vi "Target Detection.vi"(0 "Camera Image":T1) -> ()   [LabVIEW 2013]
uses:
  Support/TargetType.ctl
  <vilib>/vision/Image Controls.llb/IMAQ Image.ctl
  Robot Global Data.vi
panel:
  out "loop time ms":u32
  in  "Instructions:":string="Images:\nUse the tab immediately below to choose the image source. Update the camera settings or the image directory so that you have images or video to test with.\n\nCalibration:\nYou can update Color Component ranges directly, or by clicking and drawing a line on the colored strip in the Image control. The Std Dev multipliers and where the strip is drawn determine the calibration values.\n\nUse Debugging tab to view the result of the color range threshold .\n\nArea Size LImit is used to ignore objects too small or far away to care about.\n\nThe Details tab contains score details for each target and subObject.\n\nCamera Type is used to select lens angles for distance calculation.\n\nVertical strips with no adjacent horizontal strip are identified as \"not hot\" and marked in blue.\nThe numeric scores indicate represent aspect ratio and rectangularity.\n\nWhen both strips are near enough, the pair is identified as \"hot\" and marked in green. Scores\nindicate the left, right, ratio of widths, and vertical positioning.\n\nAny score that falls below cutoff is drawn in red and bounding box is drawn in red."
  in  "Std Devs":cluster{"Hue":dbl, "Sat":dbl, "Val":dbl}={"Hue"=4.0, "Sat"=6.0, "Val"=4.0}
  in  "Area Size Limit %":dbl=0.06 format="%#_13g"
  in  "Camera Type":enum16{"206", "1011", "1013"}(ring)=enum."1013"
  in  "Score Cutoff":dbl(slide)=54.248366013071895 scale=0.0..100.0
  in  "Color Components":T2={"Hue"={112.0, 144.0}, "Sat"={223.0, 255.0}, "Val"={237.0, 255.0}} {"Val" scale=0.0..255.0; "Sat" scale=0.0..255.0; "Hue" scale=0.0..255.0 scale format="%#_3g"}
  in  "Tabbed Info":enum32{"Debugging", "Details"}(tab)=enum."Details"
  out "Mask":T1(plugin-control)
  out "Target Info":T4(array[cluster])=[{"Scores"={"Total"=264.8428070737725, "Left"=82.00744831503384, "Right"=0.0, "Ratio"=95.56961423095669, "Vertical"=87.265744527782, "index"=0, "State"=enum."Hot"}, "Verticals"={"Horizontal?"=FALSE, "Aspect Score"=83.06845793962944, "Rect Score"=72.28571428571429, {"Left"=200.0, "Top"=96.0, "Right"=207.0, "Bottom"=146.0}, "Equiv H"=5.125465815260874, "Equiv V"=49.36136716524427}, "Horizontals"={"Horizontal?"=TRUE, "Aspect Score"=88.35576607935369, "Rect Score"=66.38655462184875, {"Left"=161.0, "Top"=90.0, "Right"=195.0, "Bottom"=97.0}, "Equiv H"=32.1921978337671, "Equiv V"=4.908021527945207}, "Distance ft"=14.225212029119403, "Center"={"X"=0.271875, "Y"=0.008333333333333333}}]
  out "Image":T1(plugin-control)
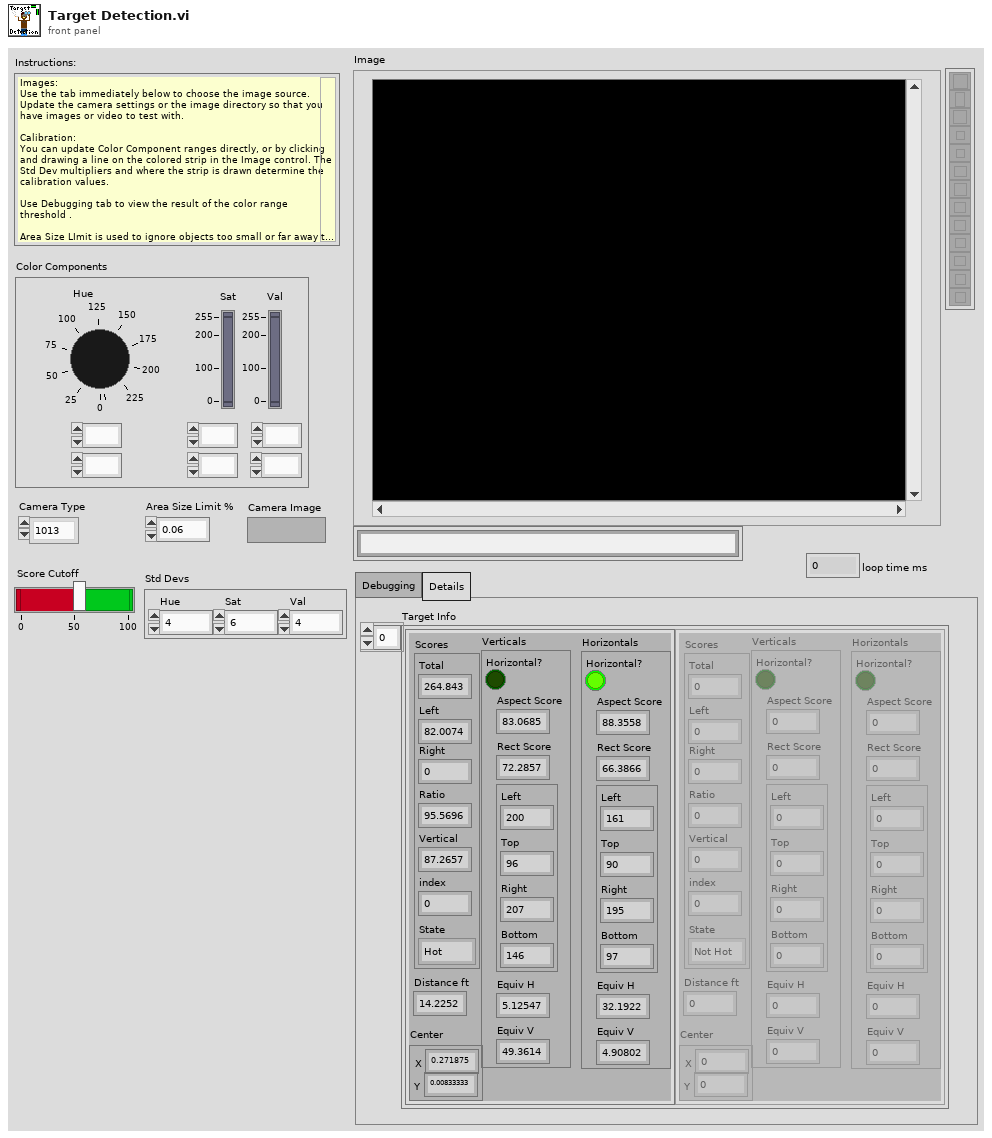
[diagram p1: front panel]
types:
  T1 = typedef "IMAQ Image.ctl" = refnum<image>
  T2 = cluster{"Hue":cluster{dbl, dbl}, "Sat":cluster{dbl, dbl}, "Val":cluster{dbl, dbl}}
  T3 = typedef "TargetType.ctl" = enum16{"Not Hot", "Hot"}
  T4 = cluster{"Scores":cluster{"Total":dbl, "Left":dbl, "Right":dbl, "Ratio":dbl, "Vertical":dbl, "index":i32, "State":T3}, "Verticals":cluster{"Horizontal?":bool, "Aspect Score":dbl, "Rect Score":dbl, cluster{"Left":dbl, "Top":dbl, "Right":dbl, "Bottom":dbl}, "Equiv H":dbl, "Equiv V":dbl}, "Horizontals":cluster{"Horizontal?":bool, "Aspect Score":dbl, "Rect Score":dbl, cluster{"Left":dbl, "Top":dbl, "Right":dbl, "Bottom":dbl}, "Equiv H":dbl, "Equiv V":dbl}, "Distance ft":dbl, "Center":cluster{"X":dbl, "Y":dbl}}[]
  T5 = cluster{"Horizontal":bool, "Aspect Score":dbl, "Rect Score":dbl, cluster{"Left":dbl, "Top":dbl, "Right":dbl, "Bottom":dbl}, "Equiv H":dbl, "Equiv V":dbl}[]
  T6 = cluster{cluster{dbl, dbl}, cluster{dbl, dbl}, cluster{dbl, dbl}}
  T7 = cluster{"Scores":cluster{"Total":dbl, "Left":dbl, "Right":dbl, "Ratio":dbl, "Vertical":dbl, "index":i32, "State":T3}, "Verticals":cluster{"Horizontal?":bool, "Aspect Score":dbl, "Rect Score":dbl, cluster{"Left":dbl, "Top":dbl, "Right":dbl, "Bottom":dbl}, "Equiv H":dbl, "Equiv V":dbl}, "Horizontals":cluster{"Horizontal?":bool, "Aspect Score":dbl, "Rect Score":dbl, cluster{"Left":dbl, "Top":dbl, "Right":dbl, "Bottom":dbl}, "Equiv H":dbl, "Equiv V":dbl}, "Validated":bool}[]
  T8 = cluster{"Scores":cluster{"Total":dbl, "Left":dbl, "Right":dbl, "Ratio":dbl, "Vertical":dbl, "index":i32, "State":T3}, "Verticals":cluster{"Horizontal?":bool, "Aspect Score":dbl, "Rect Score":dbl, cluster{"Left":dbl, "Top":dbl, "Right":dbl, "Bottom":dbl}, "Equiv H":dbl, "Equiv V":dbl}, "Horizontals":cluster{"Horizontal?":bool, "Aspect Score":dbl, "Rect Score":dbl, cluster{"Left":dbl, "Top":dbl, "Right":dbl, "Bottom":dbl}, "Equiv H":dbl, "Equiv V":dbl}, "Distance (ft)":dbl, "Target Center (-1 to 1)":cluster{"X":dbl, "Y":dbl}}[]
  T9 = cluster{"Scores":cluster{"Total":dbl, "Left":dbl, "Right":dbl, "Ratio":dbl, "Vertical":dbl, "index":i32, "State":T3}, "Verticals":cluster{"Horizontal?":bool, "Aspect Score":dbl, "Rect Score":dbl, cluster{"Left":dbl, "Top":dbl, "Right":dbl, "Bottom":dbl}, "Equiv H":dbl, "Equiv V":dbl}, "Horizontals":cluster{"Horizontal?":bool, "Aspect Score":dbl, "Rect Score":dbl, cluster{"Left":dbl, "Top":dbl, "Right":dbl, "Bottom":dbl}, "Equiv H":dbl, "Equiv V":dbl}, "Distance (ft)":dbl, "Target Center (-1 to 1)":cluster{"X":dbl, "Y":dbl}}
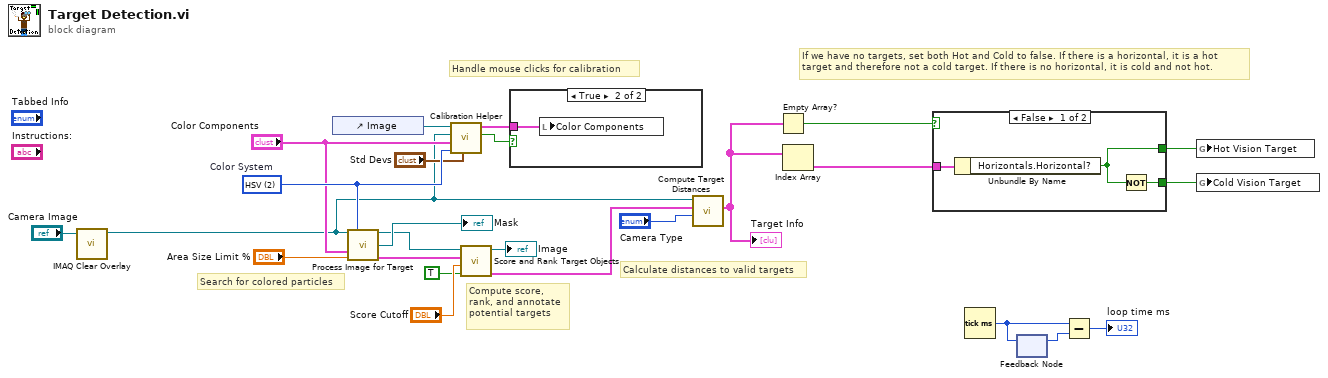
[diagram p0: block diagram]
diagram:
  w16 = u16 2 items=["RGB", "HSL", "HSV", "HSI"]  # Color System
  # "If we have no targets, set both Hot and Cold to false. If there is a horizontal, it is a hot\ntarget and therefore not a cold target. If there is no horizontal, it is cold and not hot."
  # "Calculate distances to valid targets"
  # "Search for colored particles"
  # "Handle mouse clicks for calibration"
  # "Compute score,\nrank, and annotate\npotential targets"
  n1 = call "IMAQ Clear Overlay"("Image"="Camera Image") -> ("Image Out"=w11:T1)  [unwired: 9 in, 1 out]
  n2 = control-ref of="Image"() -> (w17:refnum<vi>)
  n3 = call "Process Image for Target.vi"("Src Image"=w11, "Color Mode"=w16, "Color Components"="Color Components", "Area Cutoff %"="Area Size Limit %") -> ("Src Image Out"=w23:T1, "Threshold"=→"Mask":T1, "Particles"=w20:T5)  [unwired: 9 in]
  n4 = call "Calibration Helper.vi"("Std Devs"="Std Devs", "Color Mode"=w16, "Color Components"="Color Components", "Image"=w11, "Image Ctl Refnum"=w17) -> ("Changed"=w12:bool, "output color"=w14:T6)  [unwired: 5 in]
  n5 = call "Score and Rank Target Objects.vi"("Annotate"=TRUE, "Score Limit"="Score Cutoff", "Particles"=w20, "Image in"=w23) -> ("Target Info"=w19:T7, "Annotated Image"=→"Image":T1)  [unwired: 6 in]
  n6 = case shown="True" w12 {
    tunnel: w14 -> [_ w26]
    frame False {
    }
    frame True {
      n7 = local write "Color Components"(w26) -> ()
    }
  }
  n8 = call "Compute Target Distances.vi"("Camera Type"="Camera Type", "Target Info"=w19, "Image in"=w11) -> ("Target Info"=w4:T8)  [unwired: 6 in, 2 out]
  "Target Info" <- w4
  n9 = Empty Array?(array=w4) -> (empty?=w5:bool)
  n10 = Index Array(array=w4) -> (element=w8:T9)  [unwired: 1 in]
  n11 = case shown="False" w5 {
    tunnel: w8 -> [w29 _]
    tunnel: [w28 _] -> w7
    tunnel: [w27 _] -> w6
    frame False {
      n12 = Unbundle By Name(w29) -> ("Horizontals.Horizontal?"=w28:bool)
      n13 = Not(x=w28) -> (.not. x?=w27:bool)
    }
    frame True {
    }
  }
  n14 = Tick Count (ms)() -> (millisecond timer value=w3:u32)
  n15 = feedback #1() -> (w2:u32)  [unwired: 1 in]
  n16 = feedback-in #1(w3) -> ()
  n17 = Subtract(x=w3, y=w2) -> (x-y=→"loop time ms":u32)
  n18 = global write "Robot Global Data.vi" "Hot Vision Target"(w7) -> ()
  n19 = global write "Robot Global Data.vi" "Cold Vision Target"(w6) -> ()
